vi "set 24C temp(SubVI).vi"(6 "Control":bool=TRUE, 8 "error in":errorcluster, 9 "Temperature":dbl, 10 "Rate":dbl, 11 "VISA引用句柄输入":refnum<visa-resource-name>) -> (0 "ErrorOut":errorcluster={"status"=TRUE, "code"=-1073807339, "source"="VISA Read in Cryocon_R/W.vi->Loop_Source.vi"})   [LabVIEW 2019, in "9T cmag.lvlib"]
uses:
  9T cmag.lvlib
  SubVI.lvlib
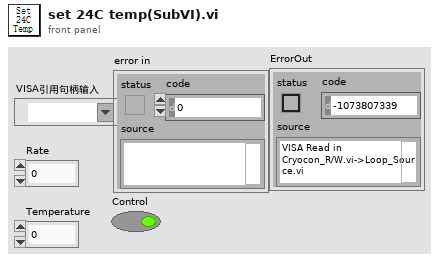
[diagram p1: front panel]
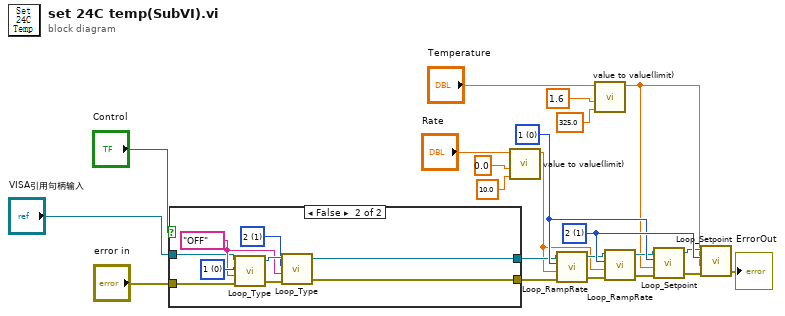
[diagram p0: block diagram]
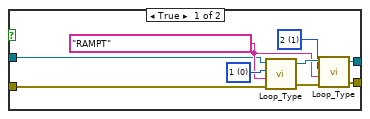
[diagram p2: hidden frame]
diagram:
  w22 = u8 1 items=["1", "2", "3", "4"] ("Loop")
  w20 = u8 0 items=["1", "2", "3", "4"] ("Loop")
  n1 = case shown="False" "Control" {
    tunnel: "VISA引用句柄输入" -> [w26 w35]
    tunnel: [w25 w34] -> w12
    tunnel: "error in" -> [w24 w33]
    tunnel: [w23 w32] -> w10
    frame True {
      w27 = "RAMPT" ("Type")
      w28 = u8 1 items=["1", "2", "3", "4"] ("Loop")
      w31 = u8 0 items=["1", "2", "3", "4"] ("Loop")
      n2 = call "Loop_Type.vi"("VISA in"=w26, "Loop"=w31, "Loop Type"=w27, "error in"=w24) -> ("VISA out"=w30:refnum<visa-resource-name>, "ErrorOut"=w29:errorcluster)  [unwired: 1 in, 1 out]
      n3 = call "Loop_Type.vi"("VISA in"=w30, "Loop"=w28, "Loop Type"=w27, "error in"=w29) -> ("VISA out"=w25:refnum<visa-resource-name>, "ErrorOut"=w23:errorcluster)  [unwired: 1 in, 1 out]
    }
    frame False {
      w36 = "OFF" ("Type")
      w37 = u8 1 items=["1", "2", "3", "4"] ("Loop")
      w40 = u8 0 items=["1", "2", "3", "4"] ("Loop")
      n4 = call "Loop_Type.vi"("VISA in"=w35, "Loop"=w40, "Loop Type"=w36, "error in"=w33) -> ("VISA out"=w39:refnum<visa-resource-name>, "ErrorOut"=w38:errorcluster)  [unwired: 1 in, 1 out]
      n5 = call "Loop_Type.vi"("VISA in"=w39, "Loop"=w37, "Loop Type"=w36, "error in"=w38) -> ("VISA out"=w34:refnum<visa-resource-name>, "ErrorOut"=w32:errorcluster)  [unwired: 1 in, 1 out]
    }
  }
  n6 = call "value to value(limit).vi"("high limit"=10.0 ("y"), "low limit"=0.0, "数值 in"="Rate") -> ("数值 out"=w1:dbl)  [unwired: 8 in]
  n7 = call "Loop_RampRate.vi"("VISA in"=w12, "Loop"=w20, "Ramp Rate (K/Min)"=w1, "error in"=w10) -> ("VISA out"=w18:refnum<visa-resource-name>, "ErrorOut"=w17:errorcluster)  [unwired: 1 in, 1 out]
  n8 = call "value to value(limit).vi"("high limit"=325.0 ("y"), "low limit"=1.6, "数值 in"="Temperature") -> ("数值 out"=w5:dbl)  [unwired: 8 in]
  n9 = call "Loop_RampRate.vi"("VISA in"=w18, "Loop"=w22, "Ramp Rate (K/Min)"=w1, "error in"=w17) -> ("VISA out"=w19:refnum<visa-resource-name>, "ErrorOut"=w16:errorcluster)  [unwired: 1 in, 1 out]
  n10 = call "Loop_Setpoint.vi"("VISA in"=w19, "Loop"=w20, "Setpoint"=w5, "error in"=w16) -> ("VISA out"=w21:refnum<visa-resource-name>, "ErrorOut"=w15:errorcluster)  [unwired: 1 in, 1 out]
  n11 = call "Loop_Setpoint.vi"("VISA in"=w21, "Loop"=w22, "Setpoint"=w5, "error in"=w15) -> ("ErrorOut"=→"ErrorOut":errorcluster)  [unwired: 1 in, 2 out]
